vi "Update DemoService.vi"(8 "error in (no error)":errorcluster, 10 "DemoService":i32=-2, 11 "DIMDemoServer in":refnum<class "DIMDemoServer.lvclass">) -> (0 "error out":errorcluster, 3 "DIMDemoServer out":refnum<class "DIMDemoServer.lvclass">)   [LabVIEW 2012, in "DimActorDemo.lvlib" / "DIMDemoServer.lvclass"]
uses:
  DIMDemoServer.lvclass
  DIMActor/DIMActor/DIMActor.lvclass/DIMActor.ctl
  DIMActor/DIMActor/DIMActor.lvclass
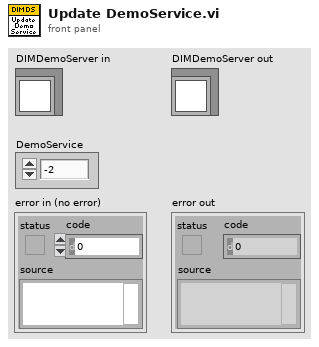
[diagram p1: front panel]
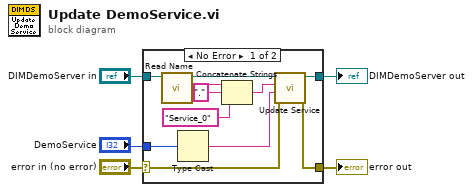
[diagram p0: block diagram]
diagram:
  n1 = case shown="No Error" "error in (no error)" {
    selector: "error in (no error)" -> [w13 w18]
    tunnel: [w12 w18] -> w4
    tunnel: [w16 w17] -> w2
    tunnel: "DIMDemoServer in" -> [w8 w17]
    tunnel: "DemoService" -> [w15 _]
    frame No Error {
      n2 = call "Read Name.vi"("DIMActor in"=w8) -> ("Name"=w6:string, "DIMActor out"=w7:refnum<class "DIMDemoServer.lvclass">)  [unwired: 8 in, 1 out]
      n3 = Type Cast(x=w15) -> (*(type *) &x=w14:string)  [unwired: 1 in]
      n4 = Concatenate Strings(w6, "." ("string"), "Service_0" ("Service Name")) -> (w9:string)
      n5 = call "Update Service.vi"("error in (no error)"=w13, "data"=w14, "Service Name"=w9, "DIMActor in"=w7) -> ("error out"=w12:errorcluster, "DIMActor out"=w16:refnum<class "DIMDemoServer.lvclass">)  [unwired: 6 in]
    }
    frame Error {
    }
  }
  "error out" <- w4
  "DIMDemoServer out" <- w2
